vi "Show DB.vi"() -> (3 "Result Set":string[][](table) caption="Database Albums")   [LabVIEW 2015]
doc: "Shows the contents of the database."
uses:
  <vilib>/drjdpowell/SQLite Library/SQL Connection/Open (string).vi
  <vilib>/drjdpowell/SQLite Library/SQL Connection/Connection.lvclass
panel:
  out "error out":errorcluster
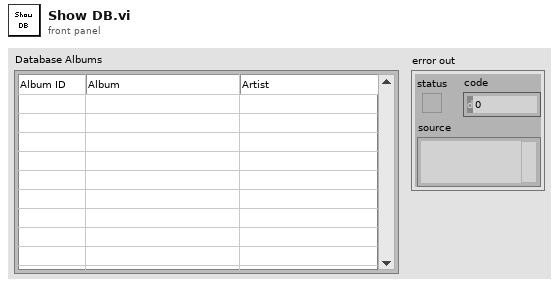
[diagram p1: front panel]
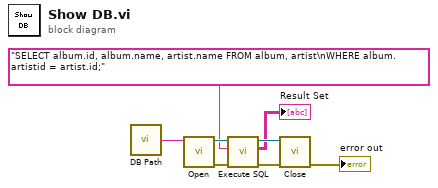
[diagram p0: block diagram]
diagram:
  n1 = call "DB Path.vi"() -> ("DB Path"=w8:string)
  n2 = call-poly <vilib>:"Open.vi"("db file"=w8) -> ("error out"=w4:errorcluster, "SQLite Connection"=w5:refnum<class "Connection.lvclass">)  [unwired: 9 in]
  n3 = call <vilib>:"Execute SQL.vi"("error in (no error)"=w4, "SQL"="SELECT album.id, album.name, artist.name FROM album, artist\nWHERE album.artistid = artist.id;", "SQLite Connection in"=w5) -> ("error out"=w6:errorcluster, "Result Set"=→"Result Set":string[][], "SQLite Connection"=w7:refnum<class "Connection.lvclass">)  [unwired: 5 in, 1 out]
  n4 = call-dynamic "Close.vi"("error in (no error)"=w6, "SQLite Connection in"=w7) -> ("error out"=→"error out":errorcluster)  [unwired: 9 in]
